vi "PicoScope3000aGetEts.vi"(0 "error in":errorcluster, 2 "handle in":i16, 3 "Acquisition Settings":T4 {"Down Sample Ratio" min=1 step=1; "Down-Sample Mode" items=["None", "Aggregate", "Decimate", "Average"]}, 8 "Device Info":T1) -> (1 "time array":i64[](array[numeric]), 4 "overflow":i16, 5 "noOfSamples":u32, 6 "error out":errorcluster, 7 "handle out":i16, 9 "Buffers (Max or non-aggregated)":T3, 10 "Min Buffers":T2)   [LabVIEW 2009]
doc: "This VI collects a block of data from the oscilloscope. This can be called in a loop in order to continually collect blocks of data. The oscilloscope should first be set up by using PicoScope3000aSettings.vi. The VI outputs data arrays in two clusters (max and min). If not using aggregation, 'Min Buffers' is not used."
uses:
  ps3000a.dll
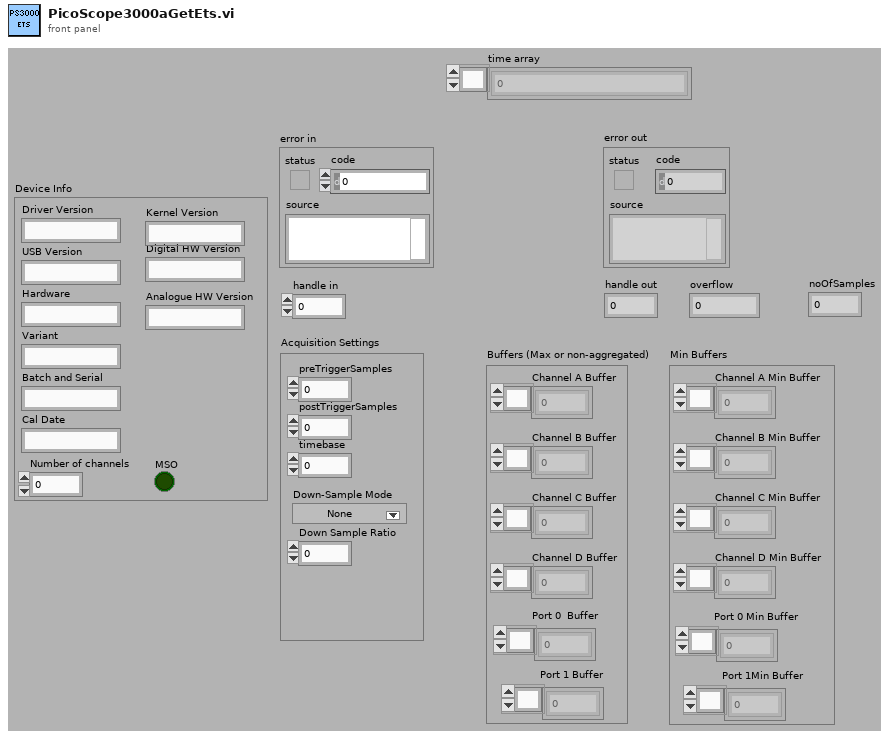
[diagram p1: front panel]
types:
  T1 = cluster{"Driver Version":string, "USB Version":string, "Hardware":string, "Variant":string, "Batch and Serial":string, "Cal Date":string, "Kernel Version":string, "Digital HW Version":string, "Analogue HW Version":string, "MSO":bool, "Number of channels":i16}
  T2 = cluster{"Channel A Min Buffer":i16[], "Channel B Min Buffer":i16[], "Channel C Min Buffer":i16[], "Channel D Min Buffer":i16[], "Port 0 Min Buffer ":i16[], "Port 1Min Buffer ":i16[]}
  T3 = cluster{"Channel D Buffer":i16[], "Channel C Buffer":i16[], "Channel B Buffer":i16[], "Channel A Buffer":i16[], "Port 0  Buffer ":i16[], "Port 1 Buffer ":i16[]}
  T4 = cluster{"preTriggerSamples":u32, "postTriggerSamples":u32, "timebase":u32, "Down-Sample Mode":i32, "Down Sample Ratio":u32}
  T5 = cluster{"Channel A Min Buffer":i16[], "Channel B Min Buffer":i16[], "Channel C Min Buffer":i16[], "Channel D Min Buffer":i16[], "Port 0 Min Buffer":i32[], "Port 1 Min Buffer":i32[]}
  T6 = cluster{"Channel D Buffer":i16[], "Channel C Buffer":i16[], "Channel B Buffer":i16[], "Channel A Buffer":i16[], "Port 0 Max Buffer":i32[], "Port 1 Max Buffer":i32[]}
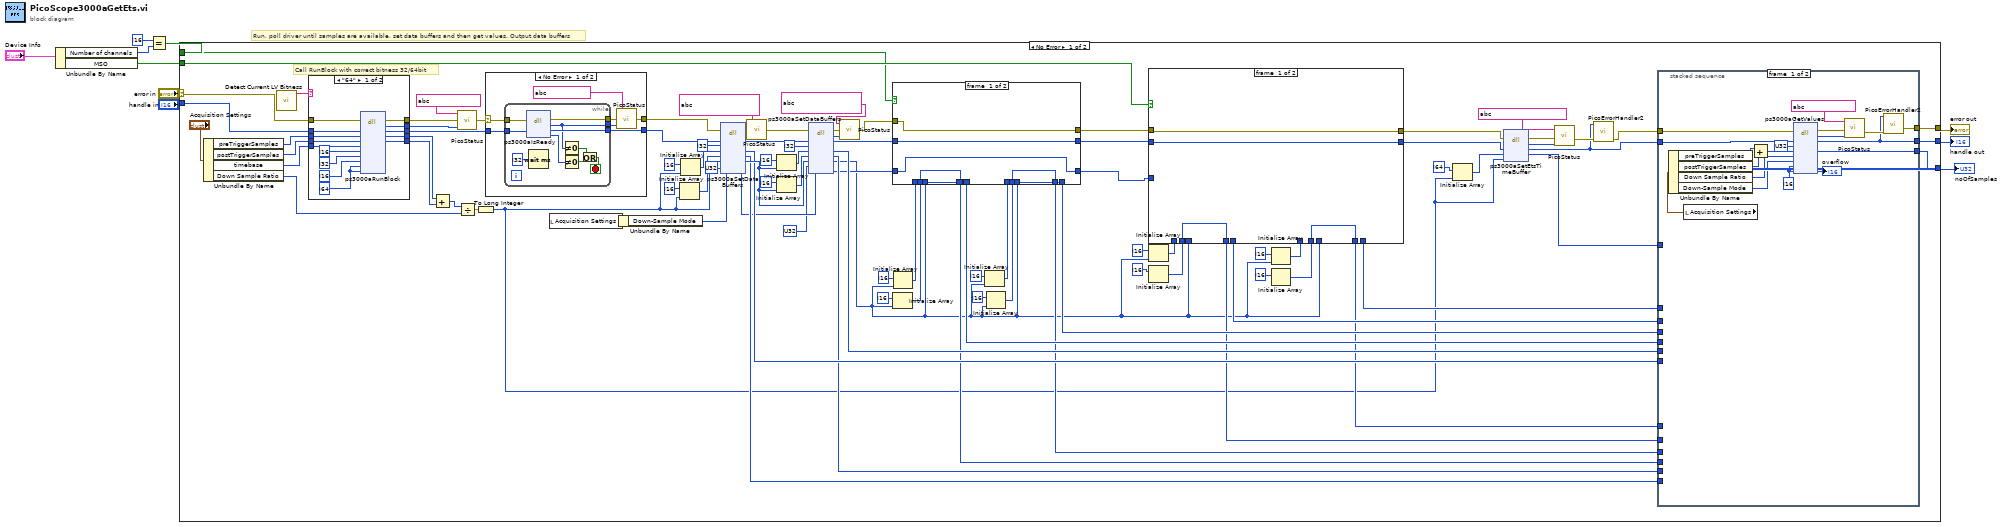
[diagram p0: block diagram]
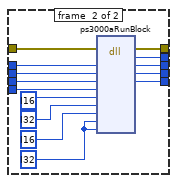
[diagram p2: hidden frame]
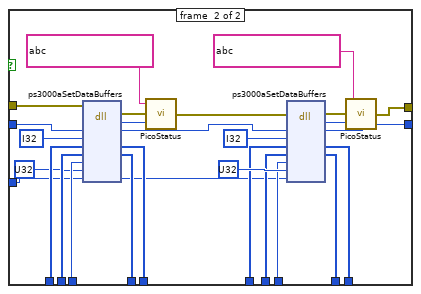
[diagram p3: hidden frame]
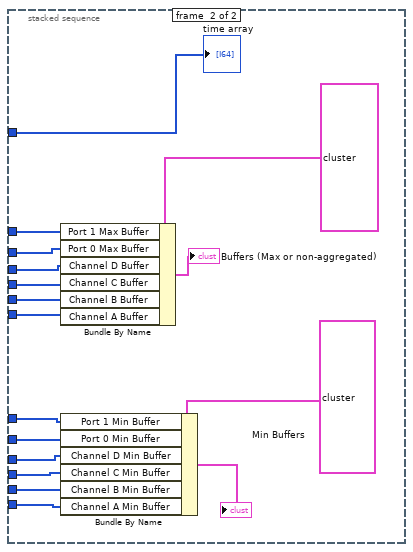
[diagram p4: hidden frame]
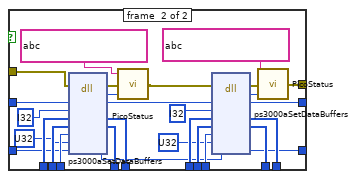
[diagram p6: hidden frame]
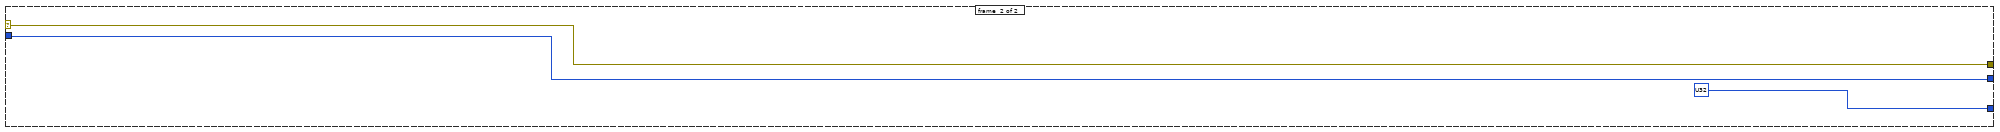
[diagram p7: hidden frame]
diagram:
  # "Run, poll driver until samples are available, set data buffers and then get values. Output data buffers"
  n1 = Unbundle By Name("Device Info") -> ("Number of channels"=w4:i16, "MSO"=w3:bool)
  n2 = Equal?(x=i16 ?, y=w4) -> (x = y?=w2:bool)
  n3 = case shown="No Error" "error in" {
    selector: "error in" -> [w16 w258]
    tunnel: [w84 w258] -> w9
    tunnel: "handle in" -> [w15 w257]
    tunnel: [w83 w257] -> w7
    tunnel: [w40 u32 ? ("noOfSamples")] -> w6
    tunnel: w3 -> [w39 _]
    tunnel: w2 -> [w38 _]
    frame #0 {
      # "Call RunBlock with correct bitness 32/64bit"
      n4 = Unbundle By Name("Acquisition Settings") -> ("preTriggerSamples"=w14:u32, "postTriggerSamples"=w13:u32, "timebase"=w12:u32, "Down Sample Ratio"=w11:u32)
      n5 = call "Detect Current LV Bitness.vi"() -> ("bitness"=w20:string)  [unwired: 11 in]
      n6 = case shown="\"64\"" w20 {
        tunnel: [w119 w133] -> w18
        tunnel: [w118 w132] -> w25
        tunnel: [w117 w131] -> w24
        tunnel: w12 -> [w116 w130]
        tunnel: w14 -> [w115 w129]
        tunnel: w13 -> [w114 w128]
        tunnel: [w113 w127] -> w23
        tunnel: [w112 w126] -> w22
        tunnel: w16 -> [w111 w125]
        tunnel: w15 -> [w110 w124]
        frame #0 {
          w106 = i64 ? ("pParameter")
          n7 = dll-call lib="ps3000a.dll" fn="ps3000aRunBlock" ("ps3000.dll:_ps3000_open_unit@0")(error in=w111, "handle"=w110, "preTriggerSamples"=w115, "postTriggerSamples"=w114, "timebase"=w116, "oversample"=i16 ?, "timeindisposed"=i32 ? ("pParameter"), "segmentIndex"=i16 ? ("pParameter"), "lpReady"=w106, "pParameter"=w106) -> (error out=w112:errorcluster, "PICO_STATUS"=w113:i32, "handle"=w119:i16, "preTriggerSamples"=w118:u32, "postTriggerSamples"=w117:u32)  [unwired: 8 in, 1 out]
        }
        frame #1 {
          w120 = i32 ? ("pParameter")
          n8 = dll-call lib="ps3000a.dll" fn="ps3000aRunBlock" ("ps3000.dll:_ps3000_open_unit@0")(error in=w125, "handle"=w124, "preTriggerSamples"=w129, "postTriggerSamples"=w128, "timebase"=w130, "oversample"=i16 ?, "timeindisposed"=i32 ? ("pParameter"), "segmentIndex"=i16 ? ("pParameter"), "lpReady"=w120, "pParameter"=w120) -> (error out=w126:errorcluster, "PICO_STATUS"=w127:i32, "handle"=w133:i16, "preTriggerSamples"=w132:u32, "postTriggerSamples"=w131:u32)  [unwired: 8 in, 1 out]
        }
      }
      n9 = Add(x=w25, y=w24) -> (x+y=w17:u32)
      n10 = call "PicoStatus.vi"("PICO STATUS"=w23, "error in"=w22, "source"=string ?) -> ("error out"=w19:errorcluster)
      n11 = Divide(x=w17, y=w11) -> (x/y=w63:dbl)
      n12 = To Long Integer(number=w63) -> (32bit integer=w28:i32)
      n13 = case shown="No Error" w19 {
        selector: w19 -> [w206 w219]
        tunnel: [w207 w218] -> w105
        tunnel: [w205 w219] -> w95
        tunnel: w18 -> [w201 w218]
        frame #0 {
          n14 = while {
            tunnel: [w217] -> w207
            tunnel: [w212] -> w203
            tunnel: w206 -> [w211]
            tunnel: [w210] -> w204
            tunnel: w201 -> [w208]
            stop <- w216 stop-if-true
            n15 = dll-call lib="ps3000a.dll" fn="ps3000aIsReady" ("ps3000.dll:_ps3000_open_unit@0")(error in=w211, "handle"=w208) -> (error out=w210:errorcluster, "status"=w212:u32, "handle"=w217:i16, "ready"=w213:i16)  [unwired: 3 in, 1 out]
            n16 = Wait (ms)(milliseconds to wait=i32 ?) -> ()  [unwired: 1 out]
            n17 = Not Equal To 0?(x=w212) -> (x != 0?=w214:bool)
            n18 = Not Equal To 0?(x=w213) -> (x != 0?=w215:bool)
            n19 = Or(x=w214, y=w215) -> (x .or. y?=w216:bool)
          }
          n20 = call "PicoStatus.vi"("PICO STATUS"=w203, "error in"=w204, "source"=string ?) -> ("error out"=w205:errorcluster)
        }
        frame #1 {
        }
      }
      n21 = local read "Acquisition Settings"() -> (w62:T4)
      n22 = Unbundle By Name(w62) -> ("Down-Sample Mode"=w60:i32)
      n23 = Initialize Array(i16 ? ("element"), w28) -> (w81:i16[])
      n24 = Initialize Array(i16 ? ("element"), w28) -> (w102:i16[])
      n25 = dll-call lib="ps3000a.dll" fn="ps3000aSetDataBuffers" ("ps3000.dll:_ps3000_open_unit@0")(error in=w95, "handle"=w105, "channel"=i32 ?, "bufferMax"=w102, "bufferMin"=w81, "bufferLth"=w28, "segmentIndex"=u32 ?, "mode"=w60) -> (error out=w91:errorcluster, "PICO_STATUS"=w92:u32, "handle"=w104:i16, "bufferMax"=w68:i16[], "bufferMin"=w64:i16[], "bufferLth"=w72:i32, "mode"=w59:i32)  [unwired: 4 in, 1 out]
      n26 = call "PicoStatus.vi"("PICO STATUS"=w92, "error in"=w91, "source"=string ?) -> ("error out"=w90:errorcluster)
      n27 = Initialize Array(i16 ? ("element"), w72) -> (w99:i16[])
      n28 = Initialize Array(i16 ? ("element"), w72) -> (w79:i16[])
      n29 = dll-call lib="ps3000a.dll" fn="ps3000aSetDataBuffers" ("ps3000.dll:_ps3000_open_unit@0")(error in=w90, "handle"=w104, "channel"=i32 ?, "bufferMax"=w99, "bufferMin"=w79, "bufferLth"=w72, "segmentIndex"=u32 ?, "mode"=w59) -> (error out=w88:errorcluster, "PICO_STATUS"=w89:i32, "handle"=w103:i16, "bufferMax"=w69:i16[], "bufferMin"=w65:i16[], "bufferLth"=w41:i32, "mode"=w58:i32)  [unwired: 4 in, 1 out]
      n30 = call "PicoStatus.vi"("PICO STATUS"=w89, "error in"=w88, "source"=string ?) -> ("error out"=w87:errorcluster)
      n31 = Initialize Array(i16 ? ("element"), w41) -> (w76:i16[])
      n32 = Initialize Array(i16 ? ("element"), w41) -> (w98:i16[])
      n33 = Initialize Array(i16 ? ("element"), w41) -> (w97:i16[])
      n34 = Initialize Array(i16 ? ("element"), w41) -> (w73:i16[])
      n35 = case shown="True" w38 {
        tunnel: w103 -> [w224 w255]
        tunnel: [w224 w253] -> w47
        tunnel: w98 -> [w226 w252]
        tunnel: w97 -> [w225 w251]
        tunnel: [w225 w250] -> w71
        tunnel: [w226 w249] -> w70
        tunnel: w87 -> [w223 w246]
        tunnel: [w223 w240] -> w48
        tunnel: w76 -> [w222 w237]
        tunnel: w73 -> [w221 w236]
        tunnel: [w221 w235] -> w67
        tunnel: [w222 w234] -> w66
        tunnel: w41 -> [_ w233]
        tunnel: w41 -> [_ w232]
        tunnel: w58 -> [w220 w231]
        tunnel: [w220 w227] -> w46
        frame #0 {
        }
        frame #1 {
          n36 = dll-call lib="ps3000a.dll" fn="ps3000aSetDataBuffers" ("ps3000.dll:_ps3000_open_unit@0")(error in=w246, "handle"=w255, "channel"=i32 ?, "bufferMax"=w252, "bufferMin"=w237, "bufferLth"=w233, "segmentIndex"=u32 ?, "mode"=w231) -> (error out=w244:errorcluster, "PICO_STATUS"=w245:i32, "handle"=w254:i16, "bufferMax"=w249:i16[], "bufferMin"=w234:i16[], "mode"=w230:i32)  [unwired: 5 in, 1 out]
          n37 = call "PicoStatus.vi"("PICO STATUS"=w245, "error in"=w244, "source"=string ?) -> ("error out"=w243:errorcluster)
          n38 = dll-call lib="ps3000a.dll" fn="ps3000aSetDataBuffers" ("ps3000.dll:_ps3000_open_unit@0")(error in=w243, "handle"=w254, "channel"=i32 ?, "bufferMax"=w251, "bufferMin"=w236, "bufferLth"=w232, "segmentIndex"=u32 ?, "mode"=w230) -> (error out=w241:errorcluster, "PICO_STATUS"=w242:i32, "handle"=w253:i16, "bufferMax"=w250:i16[], "bufferMin"=w235:i16[], "mode"=w227:i32)  [unwired: 5 in, 1 out]
          n39 = call "PicoStatus.vi"("PICO STATUS"=w242, "error in"=w241, "source"=string ?) -> ("error out"=w240:errorcluster)
        }
      }
      n40 = Initialize Array(i16 ? ("element"), w41) -> (w54:i16[])
      n41 = Initialize Array(i16 ? ("element")) -> (w53:i16[])  [unwired: 1 in]
      n42 = Initialize Array(i16 ? ("element"), w41) -> (w49:i16[])
      n43 = Initialize Array(i16 ? ("element")) -> (w50:i16[])  [unwired: 1 in]
      n44 = case shown="True" w39 {
        tunnel: w48 -> [w135 w165]
        tunnel: w47 -> [w134 w164]
        tunnel: w54 -> [_ w162]
        tunnel: w53 -> [w137 w161]
        tunnel: w41 -> [_ w160]
        tunnel: w41 -> [_ w154]
        tunnel: w50 -> [w136 w155]
        tunnel: w49 -> [_ w156]
        tunnel: [w137 w153] -> w42
        tunnel: [_ w152] -> w44
        tunnel: [w136 w151] -> w43
        tunnel: [_ w150] -> w45
        tunnel: [w134 w144] -> w33
        tunnel: [w135 w143] -> w34
        tunnel: w46 -> [_ w141]
        frame #0 {
        }
        frame #1 {
          n45 = dll-call lib="ps3000a.dll" fn="ps3000aSetDataBuffers" ("ps3000.dll:_ps3000_open_unit@0")(error in=w165, "handle"=w164, "channel"=i32 ?, "bufferMax"=w162, "bufferMin"=w161, "bufferLth"=w160, "segmentIndex"=u32 ?, "mode"=w141) -> (error out=w148:errorcluster, "PICO_STATUS"=w149:i32, "handle"=w142:i16, "bufferMax"=w152:i16[], "bufferMin"=w153:i16[], "mode"=w140:i32)  [unwired: 5 in, 1 out]
          n46 = call "PicoStatus.vi"("PICO STATUS"=w149, "error in"=w148, "source"=string ?) -> ("error out"=w145:errorcluster)
          n47 = dll-call lib="ps3000a.dll" fn="ps3000aSetDataBuffers" ("ps3000.dll:_ps3000_open_unit@0")(error in=w145, "handle"=w142, "channel"=i32 ?, "bufferMax"=w156, "bufferMin"=w155, "bufferLth"=w154, "segmentIndex"=u32 ?, "mode"=w140) -> (error out=w146:errorcluster, "PICO_STATUS"=w147:i32, "handle"=w144:i16, "bufferMax"=w150:i16[], "bufferMin"=w151:i16[])  [unwired: 6 in, 1 out]
          n48 = call "PicoStatus.vi"("PICO STATUS"=w147, "error in"=w146, "source"=string ?) -> ("error out"=w143:errorcluster)
        }
      }
      n49 = Initialize Array(i64 ? ("element"), w28) -> (w27:i64[])
      n50 = dll-call lib="ps3000a.dll" fn="ps3000aSetEtsTimeBuffer" ("ps3000.dll:_ps3000_open_unit@0")(error in=w34, "handle"=w33, "buffer"=w27, "bufferLth"=w28) -> (error out=w37:errorcluster, "PICO_STATUS"=w31:u32, "handle"=w30:i16, "buffer"=w26:i64[])  [unwired: 3 in, 1 out]
      n51 = call "PicoStatus.vi"("PICO STATUS"=w31, "error in"=w37, "source"=string ?) -> ("error out"=w35:errorcluster)
      n52 = call "PicoErrorHandler2.vi"("error in (no error)"=w35, "handle In"=w30) -> ("error out"=w32:errorcluster)  [unwired: 9 in]
      n53 = stacked-sequence {
        tunnel: w30 -> [w183 _]
        tunnel: [w177 _] -> w84
        tunnel: [w166 _] -> w83
        tunnel: w71 -> [_ w190]
        tunnel: w70 -> [_ w191]
        tunnel: w69 -> [_ w192]
        tunnel: w68 -> [_ w189]
        tunnel: w67 -> [_ w196]
        tunnel: w66 -> [_ w195]
        tunnel: w65 -> [_ w194]
        tunnel: w64 -> [_ w193]
        tunnel: w32 -> [w169 _]
        tunnel: w45 -> [_ w188]
        tunnel: w44 -> [_ w187]
        tunnel: w43 -> [_ w186]
        tunnel: w42 -> [_ w185]
        tunnel: [w168 _] -> w40
        tunnel: w26 -> [_ w184]
        frame #0 {
          w181 = i16 ? ("overflow")
          n54 = local read "Acquisition Settings"() -> (w175:T4)
          n55 = Unbundle By Name(w175) -> ("preTriggerSamples"=w172:u32, "postTriggerSamples"=w173:u32, "Down Sample Ratio"=w174:u32, "Down-Sample Mode"=w170:i32)
          n56 = Add(x=w172, y=w173) -> (x+y=w171:u32)
          n57 = dll-call lib="ps3000a.dll" fn="ps3000aGetValues" ("ps3000.dll:_ps3000_open_unit@0")(error in=w169, "handle"=w183, "startIndex"=u32 ?, "noOfSamples"=w171, "downSampleRatio"=w174, "downSampleRatioMode"=w170, "segmentIndex"=w181, "overflow"=w181) -> (error out=w180:errorcluster, "PICO_STATUS"=w167:u32, "handle"=w166:i16, "noOfSamples"=w168:u32, "overflow"=→"overflow":i16)  [unwired: 6 in, 1 out]
          n58 = call "PicoStatus.vi"("PICO STATUS"=w167, "error in"=w180, "source"=string ?) -> ("error out"=w178:errorcluster)
          n59 = call "PicoErrorHandler2.vi"("error in (no error)"=w178, "handle In"=w166) -> ("error out"=w177:errorcluster)  [unwired: 9 in]
        }
        frame #1 {
          n60 = Bundle By Name(cluster=T6 ? ("Buffers (Max or non-aggregated)"), "Port 1 Max Buffer"=w188, "Port 0 Max Buffer"=w187, "Channel D Buffer"=w190, "Channel C Buffer"=w191, "Channel B Buffer"=w192, "Channel A Buffer"=w189) -> (→"Buffers (Max or non-aggregated)":T6)
          n61 = Bundle By Name(cluster=T5 ? ("Min Buffers"), "Port 1 Min Buffer"=w186, "Port 0 Min Buffer"=w185, "Channel D Min Buffer"=w196, "Channel C Min Buffer"=w195, "Channel B Min Buffer"=w194, "Channel A Min Buffer"=w193) -> (→"Min Buffers":T5)
          "time array" <- w184
        }
      }
    }
    frame #1 {
    }
  }
  "error out" <- w9
  "handle out" <- w7
  "noOfSamples" <- w6
